vi "Olympus Control.vi"() -> ()   [LabVIEW 2018]
uses:
  lib/Olympus IX BX Series/Olympus IX BX Series.lvlib
panel:
  in  "Step (0.0 um) 2":dbl format="%.1f"
  in  "Direction (1: Down) 2":enum16{"Up", "Down"}(ring)=enum."Down"
  out "Upper Limit":dbl
  out "Lower Limit":dbl
  in  "Filter Wheel Position (1)":enum32{"", "BF", "UV", "GFP", "YFP", "RFP"}(ring)=enum."RFP"
  in  "Prism Position\n (1: Bi)":enum16{"Bi", "Side"}(ring)=enum."Side"
  in  "Objective":T1(ring)=enum."x 4"
  in  "Shutter":bool
  in  "stop":bool
  in  "Lamp Intensity [V]":dbl(slide) min=0.0 max=12.0 step=0.1 scale=0.0..12.0
  in  "Lamp Type (0: Transmitted)":enum16{"Transmitted", "Reflected"}(ring)
  in  "Enable Lamp":bool
  out "error out":errorcluster
  in  "Instrument Port":refnum<visa-resource-name>="IX2-UCB"
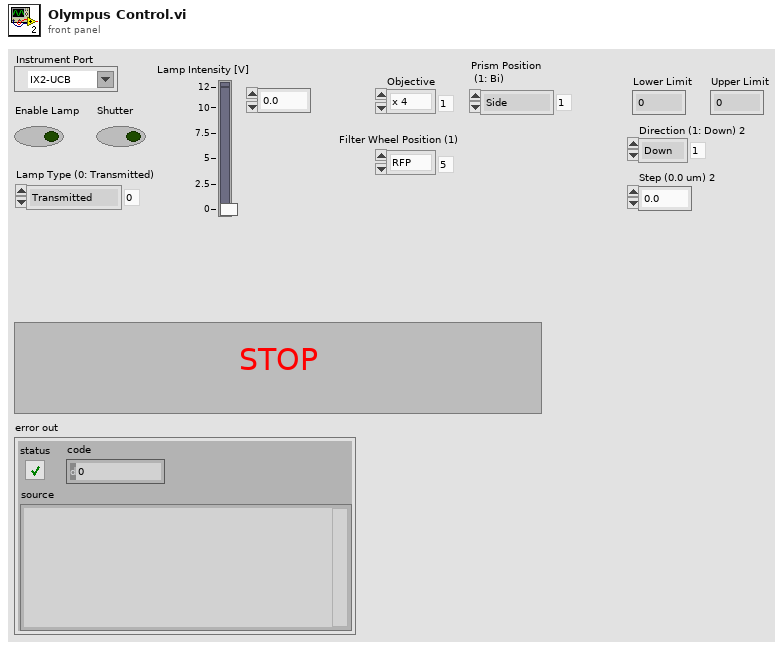
[diagram p1: front panel]
types:
  T1 = enum16{"", "x 4", "x 10", "x 20", "x 40", "x 100"}
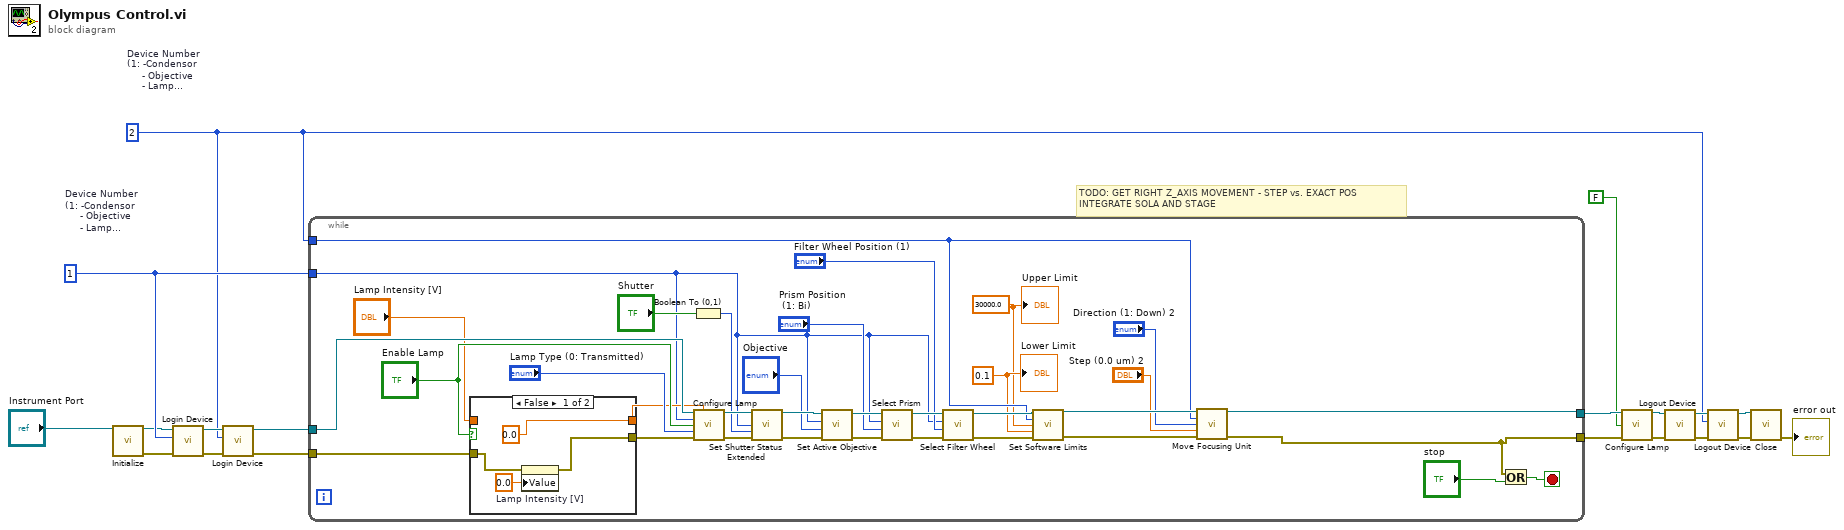
[diagram p0: block diagram]
diagram:
  w3 = 2  # Device Number (1: -Condensor      - Objective      - Lamp      - Shutter 2: - Z-Motion    - Autofocus)
  w17 = 1  # Device Number (1: -Condensor      - Objective      - Lamp      - Shutter 2: - Z-Motion    - Autofocus)
  # "TODO: GET RIGHT Z_AXIS MOVEMENT - STEP vs. EXACT POS \nINTEGRATE SOLA AND STAGE"
  n1 = call "Initialize.vi"("VISA Resource Name"="Instrument Port") -> ("VISA Resource Name Out"=w16:refnum<visa-resource-name>, "error out"=w15:errorcluster)  [unwired: 13 in]
  n2 = call "Login Device.vi"("error in (no error)"=w15, "Device Number (1)"=w17, "VISA Resource Name"=w16) -> ("error out"=w9:errorcluster, "VISA Resource Name Out"=w10:refnum<visa-resource-name>)  [unwired: 7 in]
  n3 = call "Login Device.vi"("error in (no error)"=w9, "Device Number (1)"=w3, "VISA Resource Name"=w10) -> ("error out"=w1:errorcluster, "VISA Resource Name Out"=w2:refnum<visa-resource-name>)  [unwired: 7 in]
  n4 = while {
    tunnel: w2 -> [w52]
    tunnel: w1 -> [w36]
    tunnel: [w25] -> w14
    tunnel: [w26] -> w4
    tunnel: w17 -> [w29]
    tunnel: w3 -> [w24]
    stop <- w42 stop-if-true
    w23 = 0.1 ("Far Limit (0.01 um)")
    w22 = 30000.0 ("Near Limit (30000.0 um)")
    n5 = case shown="False" "Enable Lamp" {
      tunnel: w36 -> [w57 w58]
      tunnel: [w56 w58] -> w35
      tunnel: "Lamp Intensity [V]" -> [_ w59]
      tunnel: [0.0 w59] -> w32
      frame False {
        n6 = property on="Lamp Intensity [V]" class="Slide (strict)"(error in=w57, "Value"=0.0 ("Lamp Intensity [V]")) -> (error out=w56:errorcluster)  [unwired: 1 in, 1 out]
      }
      frame True {
      }
    }
    n7 = Boolean To (0,1)(Boolean="Shutter") -> (0, 1=w48:i16)
    n8 = call "Configure Lamp.vi"("VISA Resource Name"=w52, "Lamp Intensity (1.0 V)"=w32, "Device Number (1)"=w29, "Lamp Enabled (True)"="Enable Lamp", "Lamp Type (0: Transmitted)"="Lamp Type (0: Transmitted)", "error in (no error)"=w35) -> ("VISA Resource Name Out"=w50:refnum<visa-resource-name>, "error out"=w51:errorcluster)  [unwired: 8 in]
    n9 = call "Set Shutter Status Extended.vi"("VISA Resource Name"=w50, "Shutter Control Number (1)"=w29, "Shutter Status (0: Open)"=w48, "error in (no error)"=w51) -> ("VISA Resource Name Out"=w47:refnum<visa-resource-name>, "error out"=w46:errorcluster)  [unwired: 10 in]
    n10 = call "Set Active Objective.vi"("error in (no error)"=w46, "Objective Number (1)"="Objective", "Device Number (1)"=w29, "VISA Resource Name"=w47) -> ("error out"=w43:errorcluster, "VISA Resource Name Out"=w44:refnum<visa-resource-name>)  [unwired: 6 in]
    n11 = call "Select Prism.vi"("error in (no error)"=w43, "Prism Position (0: Bi)"="Prism Position\n (1: Bi)", "Device Number (1)"=w29, "VISA Resource Name"=w44) -> ("error out"=w39:errorcluster, "VISA Resource Name Out"=w40:refnum<visa-resource-name>)  [unwired: 6 in]
    n12 = call "Select Filter Wheel.vi"("error in (no error)"=w39, "Filter Wheel Position (1)"="Filter Wheel Position (1)", "Device Number (1)"=w29, "VISA Resource Name"=w40) -> ("error out"=w30:errorcluster, "VISA Resource Name Out"=w31:refnum<visa-resource-name>)  [unwired: 6 in]
    n13 = call "Set Software Limits.vi"("VISA Resource Name"=w31, "Device Number (1)"=w24, "Near Limit (30000.0 um)"=w22, "Far Limit (0.01 um)"=w23, "error in (no error)"=w30) -> ("VISA Resource Name Out"=w28:refnum<visa-resource-name>, "error out"=w27:errorcluster)  [unwired: 9 in]
    n14 = call "Move Focusing Unit.vi"("VISA Resource Name"=w28, "Device Number (1)"=w24, "Direction (1: Down)"="Direction (1: Down) 2", "Step (0.0 um)"="Step (0.0 um) 2", "error in (no error)"=w27) -> ("VISA Resource Name Out"=w25:refnum<visa-resource-name>, "error out"=w26:errorcluster)  [unwired: 9 in]
    n15 = Or(x=w26, y="stop") -> (x .or. y?=w42:bool)
    "Lower Limit" <- w23
    "Upper Limit" <- w22
  }
  n16 = call "Configure Lamp.vi"("VISA Resource Name"=w14, "Lamp Enabled (True)"=FALSE, "error in (no error)"=w4) -> ("VISA Resource Name Out"=w13:refnum<visa-resource-name>, "error out"=w11:errorcluster)  [unwired: 11 in]
  n17 = call "Logout Device.vi"("error in (no error)"=w11, "VISA Resource Name"=w13) -> ("error out"=w7:errorcluster, "VISA Resource Name Out"=w8:refnum<visa-resource-name>)  [unwired: 8 in]
  n18 = call "Logout Device.vi"("error in (no error)"=w7, "Device Number (1)"=w3, "VISA Resource Name"=w8) -> ("error out"=w5:errorcluster, "VISA Resource Name Out"=w6:refnum<visa-resource-name>)  [unwired: 7 in]
  n19 = call "Close.vi"("VISA Resource Name"=w6, "error in (no error)"=w5) -> ("error out"=→"error out":errorcluster)  [unwired: 13 in]
